vi "FindCenterWavelength.vi"(1 "Y":dbl[](array[numeric]), 2 "X":dbl[](array[numeric])) -> (0 "CenterWaveLength":dbl)   [LabVIEW 2018]
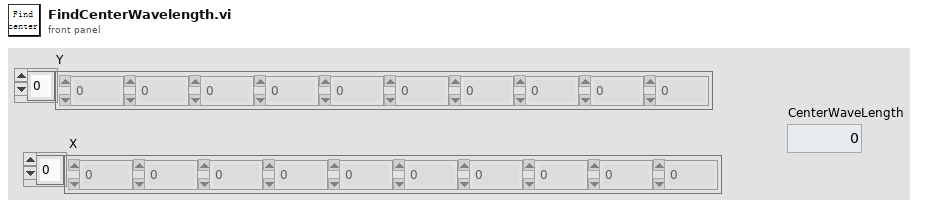
[diagram p1: front panel]
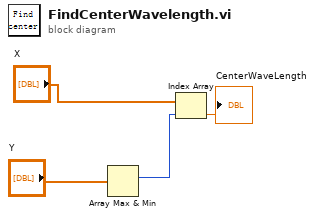
[diagram p0: block diagram]
diagram:
  n1 = Array Max & Min(array="Y") -> (max index (indices)=w2:i32)  [unwired: 3 out]
  n2 = Index Array(array="X", index=w2) -> (element=→"CenterWaveLength":dbl)
